vi "UHR-Fleezers Control (host) - 12.0_test_fpga_connection.vi"() -> ()   [LabVIEW 2014] (continued)
                                n670 = case shown="False" w1010 {
                                tunnel: w1011 -> [_ w1040]
                                tunnel: w1009 -> [w1012 _]
                                frame False {
                                n671 = flat-sequence {
                                tunnel: w1012 -> [w1013]
                                frame #0 {
                                n672 = property on="Trap Pos FB SP" class="DigNum (strict)"("Val(Sgnl)"=w1013) -> ()  [unwired: 2 in, 2 out]
                                }
                                frame #1 {
                                n673 = Wait (ms)(milliseconds to wait=u32 700) -> ()  [unwired: 1 out]
                                }
                                frame #2 {
                                n674 = local read "Action (%)"() -> (w1018:dbl)
                                n675 = Absolute Value(x=w1018) -> (abs(x)=w1017:dbl)
                                n676 = Greater?(x=w1017, y=70.0) -> (0:w1015:bool)
                                n677 = property on="Remove Action Offset" class="Bool (strict)"("Val(Sgnl)"=w1015) -> ()  [unwired: 2 in, 2 out]
                                }
                                frame #3 {
                                n678 = for {
                                N: 4 -> [_]
                                n679 = flat-sequence {
                                frame #0 {
                                n680 = Wait (ms)(milliseconds to wait=u32 500) -> ()  [unwired: 1 out]
                                }
                                frame #1 {
                                n681 = local read "Action (%)"() -> (w1024:dbl)
                                n682 = Absolute Value(x=w1024) -> (abs(x)=w1023:dbl)
                                n683 = Greater?(x=w1023, y=70.0) -> (0:w1021:bool)
                                n684 = property on="Remove Action Offset" class="Bool (strict)"("Val(Sgnl)"=w1021) -> ()  [unwired: 2 in, 2 out]
                                }
                                }
                                }
                                }
                                frame #4 {
                                n685 = Wait (ms)(milliseconds to wait=u32 500) -> ()  [unwired: 1 out]
                                }
                                frame #5 {
                                n686 = local read "Shift confocal"() -> (w1029:bool)
                                n687 = local read "Mean"() -> (w1032:dbl)
                                n688 = Greater?(x=w1032, y=11.0) -> (0:w1028:bool)
                                n689 = Not(x=w1028) -> (.not. x?=w1027:bool)
                                n690 = And(x=w1028, y=w1029) -> (x .and. y?=w1030:bool)
                                n691 = And(x=w1027, y=w1029) -> (x .and. y?=w1026:bool)
                                n692 = case shown="True" w1030 {
                                frame False {
                                }
                                frame True {
                                n693 = local read "Confocal X 2 (V)"() -> (w1035:dbl)
                                n694 = local read "Confocal Y 2 (V)"() -> (w1036:dbl)
                                n695 = property on="AO2" class="Slide (strict)"("Val(Sgnl)"=w1035) -> ()  [unwired: 2 in, 2 out]
                                n696 = property on="AO1" class="Slide (strict)"("Val(Sgnl)"=w1036) -> ()  [unwired: 2 in, 2 out]
                                }
                                }
                                n697 = case shown="True" w1026 {
                                frame False {
                                }
                                frame True {
                                n698 = local read "Confocal Y 1 (V)"() -> (w1034:dbl)
                                n699 = local read "Confocal X 1 (V)"() -> (w1033:dbl)
                                n700 = property on="AO1" class="Slide (strict)"("Val(Sgnl)"=w1034) -> ()  [unwired: 2 in, 2 out]
                                n701 = property on="AO2" class="Slide (strict)"("Val(Sgnl)"=w1033) -> ()  [unwired: 2 in, 2 out]
                                }
                                }
                                }
                                frame #6 {
                                n702 = Wait (ms)(milliseconds to wait=u32 1500) -> ()  [unwired: 1 out]
                                }
                                frame #7 {
                                n703 = property on="Remove Offset" class="Bool (strict)"("Val(Sgnl)"=TRUE ("Value (Signaling)")) -> ()  [unwired: 2 in, 2 out]
                                n704 = property on="Rem fb disp offset" class="Bool (strict)"("Val(Sgnl)"=TRUE ("Value (Signaling)")) -> ()  [unwired: 2 in, 2 out]
                                }
                                }
                                }
                                frame True {
                                n705 = flat-sequence {
                                tunnel: w1040 -> [w1041]
                                frame #0 {
                                n706 = property on="Trap D (MHz)" class="DigNum (strict)"("Val(Sgnl)"=w1041) -> ()  [unwired: 2 in, 2 out]
                                }
                                frame #1 {
                                n707 = Wait (ms)(milliseconds to wait=u32 500) -> ()  [unwired: 1 out]
                                }
                                frame #2 {
                                n708 = local read "Shift confocal"() -> (w1047:bool)
                                n709 = local read "Mean"() -> (w1048:dbl)
                                n710 = Greater?(x=w1048, y=11.0) -> (0:w1046:bool)
                                n711 = And(x=w1046, y=w1047) -> (x .and. y?=w1044:bool)
                                n712 = Not(x=w1046) -> (.not. x?=w1045:bool)
                                n713 = And(x=w1045, y=w1047) -> (x .and. y?=w1043:bool)
                                n714 = case shown="True" w1044 {
                                frame False {
                                }
                                frame True {
                                n715 = local read "Confocal Y 2 (V)"() -> (w1053:dbl)
                                n716 = local read "Confocal X 2 (V)"() -> (w1052:dbl)
                                n717 = property on="AO1" class="Slide (strict)"("Val(Sgnl)"=w1053) -> ()  [unwired: 2 in, 2 out]
                                n718 = property on="AO2" class="Slide (strict)"("Val(Sgnl)"=w1052) -> ()  [unwired: 2 in, 2 out]
                                }
                                }
                                n719 = case shown="True" w1043 {
                                frame False {
                                }
                                frame True {
                                n720 = local read "Confocal Y 1 (V)"() -> (w1051:dbl)
                                n721 = local read "Confocal X 1 (V)"() -> (w1050:dbl)
                                n722 = property on="AO2" class="Slide (strict)"("Val(Sgnl)"=w1050) -> ()  [unwired: 2 in, 2 out]
                                n723 = property on="AO1" class="Slide (strict)"("Val(Sgnl)"=w1051) -> ()  [unwired: 2 in, 2 out]
                                }
                                }
                                }
                                }
                                }
                                }
                                }
                                }
                                }
                                }
                                n724 = local read "Time (s)"() -> (w987:dbl)
                                n725 = Subtract(x=w988, y=w987) -> (x-y=w999:dbl)
                                n726 = Number To Decimal String(number=w999, width (-)=i16 0) -> (decimal integer string=w997:string)
                                n727 = Concatenate Strings(w997, " s fluorescence event") -> (w994:string)
                                n728 = local read "Messages"() -> (w995:string)
                                n729 = local write "Duration (s)"(w999) -> ()
                                n730 = call "Update messages.vi"("Message to add"=w994, "Old message string"=w995) -> ("New message string"=w993:string)
                                n731 = local write "Messages"(w993) -> ()
                                n732 = call <vilib>:"Beep.vi"() -> ()  [unwired: 12 in]
                                n733 = local write "Reset Force"(FALSE ("Force Reset")) -> ()
                                n734 = local write "Fl. High"(TRUE ("Fl. High")) -> ()
                                n735 = local write "Waiting"(TRUE ("Waiting")) -> ()
                                }
                                }
                                n736 = node-c288() -> ()  [unwired: 1 in, 1 out]
                                }
                                n737 = node-c288(w966) -> ()  [unwired: 1 out]
                                }
                              }
                            }
                          }
                          n738 = local read "Trap Pos FB SP"() -> (w875:fxp<+/-,16,1>)
                          n739 = local read "Trap D (MHz)"() -> (w877:dbl)
                        }
                      }
                    }
                    frame True {
                      n740 = flat-sequence {
                        tunnel: w1064 -> [w1074]
                        tunnel: [w1074] -> w1068
                        tunnel: w1067 -> [w1073]
                        tunnel: [w1073] -> w1066
                        tunnel: [w1072] -> w1065
                        tunnel: w1063 -> [w1071]
                        tunnel: [w1070] -> w1062
                        tunnel: w1059 -> [w1069]
                        tunnel: [w1069] -> w1058
                        tunnel: w1068 -> [w1146]
                        tunnel: w1066 -> [w1145]
                        tunnel: w1065 -> [w1144]
                        tunnel: w1062 -> [w1143]
                        tunnel: w1058 -> [w1142]
                        tunnel: [w1143] -> w1061
                        frame #0 {
                          n741 = call <vilib>:"Beep.vi"() -> ()  [unwired: 3 in, 9 out]
                          n742 = local write "Waiting"(FALSE ("Waiting")) -> ()
                          n743 = Increment(x=w1071) -> (x+1=w1070:u8)
                          n744 = case shown="\"Image\"" w1073 {
                            tunnel: w1070 -> [_ _ w1080 _]
                            frame "Image" {
                              n745 = property on="Confocal\nImage" class="Bool (strict)"("Val(Sgnl)"=TRUE ("Value (Signaling)")) -> ()  [unwired: 2 in, 2 out]
                            }
                            frame "Alarm", Default {
                            }
                            frame "Yank" {
                              n746 = flat-sequence {
                                tunnel: w1080 -> [w1083]
                                tunnel: [w1082] -> w1079
                                tunnel: ["N Array El"] -> w1078
                                tunnel: w1079 -> [w1097]
                                tunnel: w1078 -> [w1093]
                                frame #0 {
                                n747 = Multiply(x="Yank Delay (s)", y=1000.0) -> (x*y=w1086:dbl)
                                n748 = Quotient & Remainder(x=w1083, y="N Array El") -> (x-y*floor(x/y)=w1082:u8)  [unwired: 1 out]
                                n749 = Wait (ms)(milliseconds to wait=w1086) -> ()  [unwired: 1 out]
                                }
                                frame #1 {
                                n750 = Random Number (0-1)() -> (number: 0 to 1=w1094:dbl)
                                n751 = Multiply(x=w1093, y=w1094) -> (x*y=w1092:dbl)
                                n752 = Round Toward -Infinity(1:w1092) -> (0:w1091:dbl)
                                n753 = Select(t=w1091, s="Random Choice", f=w1097) -> (s? t:f=w1095:dbl)
                                n754 = Select(t="Yank to Trap D (MHz)", s="Yank to which?", f="Yank to SP") -> (s? t:f=w1088:dbl[])
                                n755 = Index Array(array=w1088, index=w1095) -> (element=w1098:dbl)
                                n756 = case shown="False" "Yank to which?" {
                                tunnel: w1098 -> [w1099 w1126]
                                frame False {
                                n757 = flat-sequence {
                                tunnel: w1099 -> [w1100]
                                frame #0 {
                                n758 = property on="Trap Pos FB SP" class="DigNum (strict)"("Val(Sgnl)"=w1100) -> ()  [unwired: 2 in, 2 out]
                                }
                                frame #1 {
                                n759 = Wait (ms)(milliseconds to wait=u32 700) -> ()  [unwired: 1 out]
                                }
                                frame #2 {
                                n760 = local read "Action (%)"() -> (w1105:dbl)
                                n761 = Absolute Value(x=w1105) -> (abs(x)=w1104:dbl)
                                n762 = Greater?(x=w1104, y=70.0) -> (0:w1102:bool)
                                n763 = property on="Remove Action Offset" class="Bool (strict)"("Val(Sgnl)"=w1102) -> ()  [unwired: 2 in, 2 out]
                                }
                                frame #3 {
                                n764 = for {
                                N: 4 -> [_]
                                n765 = flat-sequence {
                                frame #0 {
                                n766 = Wait (ms)(milliseconds to wait=u32 500) -> ()  [unwired: 1 out]
                                }
                                frame #1 {
                                n767 = local read "Action (%)"() -> (w1111:dbl)
                                n768 = Absolute Value(x=w1111) -> (abs(x)=w1110:dbl)
                                n769 = Greater?(x=w1110, y=70.0) -> (0:w1108:bool)
                                n770 = property on="Remove Action Offset" class="Bool (strict)"("Val(Sgnl)"=w1108) -> ()  [unwired: 2 in, 2 out]
                                }
                                }
                                }
                                }
                                frame #4 {
                                n771 = local read "Shift confocal"() -> (w1115:bool)
                                n772 = local read "Mean"() -> (w1118:dbl)
                                n773 = Greater?(x=w1118, y=11.0) -> (0:w1114:bool)
                                n774 = Not(x=w1114) -> (.not. x?=w1113:bool)
                                n775 = And(x=w1113, y=w1115) -> (x .and. y?=w1112:bool)
                                n776 = And(x=w1114, y=w1115) -> (x .and. y?=w1116:bool)
                                n777 = case shown="True" w1116 {
                                frame False {
                                }
                                frame True {
                                n778 = local read "Confocal X 2 (V)"() -> (w1121:dbl)
                                n779 = local read "Confocal Y 2 (V)"() -> (w1122:dbl)
                                n780 = property on="AO2" class="Slide (strict)"("Val(Sgnl)"=w1121) -> ()  [unwired: 2 in, 2 out]
                                n781 = property on="AO1" class="Slide (strict)"("Val(Sgnl)"=w1122) -> ()  [unwired: 2 in, 2 out]
                                }
                                }
                                n782 = case shown="True" w1112 {
                                frame False {
                                }
                                frame True {
                                n783 = local read "Confocal X 1 (V)"() -> (w1119:dbl)
                                n784 = local read "Confocal Y 1 (V)"() -> (w1120:dbl)
                                n785 = property on="AO1" class="Slide (strict)"("Val(Sgnl)"=w1120) -> ()  [unwired: 2 in, 2 out]
                                n786 = property on="AO2" class="Slide (strict)"("Val(Sgnl)"=w1119) -> ()  [unwired: 2 in, 2 out]
                                }
                                }
                                }
                                frame #5 {
                                n787 = Wait (ms)(milliseconds to wait=u32 1500) -> ()  [unwired: 1 out]
                                }
                                frame #6 {
                                n788 = property on="Remove Offset" class="Bool (strict)"("Val(Sgnl)"=TRUE ("Value (Signaling)")) -> ()  [unwired: 2 in, 2 out]
                                n789 = property on="Rem fb disp offset" class="Bool (strict)"("Val(Sgnl)"=TRUE ("Value (Signaling)")) -> ()  [unwired: 2 in, 2 out]
                                }
                                }
                                }
                                frame True {
                                n790 = flat-sequence {
                                tunnel: w1126 -> [w1127]
                                frame #0 {
                                n791 = property on="Trap D (MHz)" class="DigNum (strict)"("Val(Sgnl)"=w1127) -> ()  [unwired: 2 in, 2 out]
                                }
                                frame #1 {
                                n792 = Wait (ms)(milliseconds to wait=u32 500) -> ()  [unwired: 1 out]
                                }
                                frame #2 {
                                n793 = local read "Shift confocal"() -> (w1131:bool)
                                n794 = local read "Mean"() -> (w1129:dbl)
                                n795 = Greater?(x=w1129, y=11.0) -> (0:w1132:bool)
                                n796 = Not(x=w1132) -> (.not. x?=w1133:bool)
                                n797 = And(x=w1133, y=w1131) -> (x .and. y?=w1135:bool)
                                n798 = And(x=w1132, y=w1131) -> (x .and. y?=w1134:bool)
                                n799 = case shown="True" w1134 {
                                frame False {
                                }
                                frame True {
                                n800 = local read "Confocal Y 2 (V)"() -> (w1139:dbl)
                                n801 = local read "Confocal X 2 (V)"() -> (w1138:dbl)
                                n802 = property on="AO1" class="Slide (strict)"("Val(Sgnl)"=w1139) -> ()  [unwired: 2 in, 2 out]
                                n803 = property on="AO2" class="Slide (strict)"("Val(Sgnl)"=w1138) -> ()  [unwired: 2 in, 2 out]
                                }
                                }
                                n804 = case shown="True" w1135 {
                                frame False {
                                }
                                frame True {
                                n805 = local read "Confocal X 1 (V)"() -> (w1136:dbl)
                                n806 = local read "Confocal Y 1 (V)"() -> (w1137:dbl)
                                n807 = property on="AO2" class="Slide (strict)"("Val(Sgnl)"=w1136) -> ()  [unwired: 2 in, 2 out]
                                n808 = property on="AO1" class="Slide (strict)"("Val(Sgnl)"=w1137) -> ()  [unwired: 2 in, 2 out]
                                }
                                }
                                }
                                }
                                }
                                }
                                }
                              }
                            }
                            frame "Raster" {
                              n809 = property on="Trap Raster Scan" class="Bool (strict)"("Val(Sgnl)"=TRUE ("Value (Signaling)")) -> ()  [unwired: 2 in, 2 out]
                            }
                          }
                          n810 = local read "Time (s)"() -> (w1072:dbl)
                          "Fl. High" <- TRUE ("Yanking")
                        }
                        frame #1 {
                          n811 = local read "Auto F Reset"() -> (w1141:bool)
                          n812 = case shown="True" w1141 {
                            tunnel: w1146 -> [_ w1150]
                            tunnel: w1145 -> [_ w1149]
                            tunnel: w1144 -> [_ w1148]
                            tunnel: w1142 -> [_ w1147]
                            frame False {
                            }
                            frame True {
                              n813 = node-c288() -> (w1152:T26)  [unwired: 4 out]
                              n814 = timed-loop {
                                timing: w1152 -> [_]
                                timing-out: [_] -> w1151
                                tunnel: w1150 -> [w1170]
                                tunnel: w1149 -> [w1169]
                                tunnel: w1148 -> [w1168]
                                tunnel: w1147 -> [w1167]
                                stop <- w1153 stop-if-true
                                n815 = node-c288() -> ()  [unwired: 2 out]
                                n816 = local read "Fl. D Thresh. (kHz)"() -> (w1161:dbl)
                                n817 = local read "Fl. Triggered..."() -> (w1166:bool)
                                n818 = local read "Delta Fl. 1"() -> (w1157:dbl)
                                n819 = local read "Delta Fl. 2"() -> (w1155:dbl)
                                n820 = local read "Stop All"() -> (w1164:bool)
                                n821 = local read "APD to Watch"() -> (w1156:bool)
                                n822 = Select(t=w1157, s=w1156, f=w1155) -> (s? t:f=w1154:dbl)
                                n823 = Not(x=w1166) -> (.not. x?=w1165:bool)
                                n824 = Multiply(x=w1161, y=1000.0) -> (x*y=w1160:dbl)
                                n825 = Negate(x=w1160) -> (-x=w1159:dbl)
                                n826 = Less?(x=w1154, y=w1159) -> (x < y?=w1163:bool)
                                n827 = Compound Arithmetic op=OR(w1163, w1164, w1165, "Reset Force") -> (w1153:bool)
                                n828 = case shown="True" w1153 {
                                tunnel: w1170 -> [_ w1185]
                                tunnel: w1169 -> [_ w1184]
                                tunnel: w1168 -> [_ w1174]
                                tunnel: w1167 -> [_ w1176]
                                frame False {
                                }
                                frame True {
                                n829 = local read "Time (s)"() -> (w1175:dbl)
                                n830 = case shown="\"Yank\"" w1184 {
                                tunnel: w1185 -> [_ w1188]
                                tunnel: w1176 -> [_ w1186]
                                frame "Image", Default {
                                }
                                frame "Yank" {
                                n831 = flat-sequence {
                                tunnel: [w1194] -> w1189
                                tunnel: w1188 -> [w1194]
                                tunnel: [w1190] -> w1187
                                tunnel: w1186 -> [w1190]
                                tunnel: w1189 -> [w1197]
                                tunnel: w1187 -> [w1195]
                                frame #0 {
                                n832 = local read "Yank Delay (s)"() -> (w1193:dbl)
                                n833 = Multiply(x=w1193, y=1000.0) -> (x*y=w1191:dbl)
                                n834 = Wait (ms)(milliseconds to wait=w1191) -> ()  [unwired: 1 out]
                                }
                                frame #1 {
                                n835 = local read "Yank to which?"() -> (w1196:bool)
                                n836 = case shown="False" w1196 {
                                tunnel: w1197 -> [_ w1225]
                                tunnel: w1195 -> [w1198 _]
                                frame False {
                                n837 = flat-sequence {
                                tunnel: w1198 -> [w1199]
                                frame #0 {
                                n838 = property on="Trap Pos FB SP" class="DigNum (strict)"("Val(Sgnl)"=w1199) -> ()  [unwired: 2 in, 2 out]
                                }
                                frame #1 {
                                n839 = Wait (ms)(milliseconds to wait=u32 700) -> ()  [unwired: 1 out]
                                }
                                frame #2 {
                                n840 = local read "Action (%)"() -> (w1204:dbl)
                                n841 = Absolute Value(x=w1204) -> (abs(x)=w1203:dbl)
                                n842 = Greater?(x=w1203, y=70.0) -> (0:w1201:bool)
                                n843 = property on="Remove Action Offset" class="Bool (strict)"("Val(Sgnl)"=w1201) -> ()  [unwired: 2 in, 2 out]
                                }
                                frame #3 {
                                n844 = for {
                                N: 4 -> [_]
                                n845 = flat-sequence {
                                frame #0 {
                                n846 = Wait (ms)(milliseconds to wait=u32 500) -> ()  [unwired: 1 out]
                                }
                                frame #1 {
                                n847 = local read "Action (%)"() -> (w1210:dbl)
                                n848 = Absolute Value(x=w1210) -> (abs(x)=w1209:dbl)
                                n849 = Greater?(x=w1209, y=70.0) -> (0:w1207:bool)
                                n850 = property on="Remove Action Offset" class="Bool (strict)"("Val(Sgnl)"=w1207) -> ()  [unwired: 2 in, 2 out]
                                }
                                }
                                }
                                }
                                frame #4 {
                                n851 = local read "Shift confocal"() -> (w1215:bool)
                                n852 = local read "Mean"() -> (w1217:dbl)
                                n853 = Greater?(x=w1217, y=11.0) -> (0:w1214:bool)
                                n854 = Not(x=w1214) -> (.not. x?=w1213:bool)
                                n855 = And(x=w1214, y=w1215) -> (x .and. y?=w1212:bool)
                                n856 = And(x=w1213, y=w1215) -> (x .and. y?=w1211:bool)
                                n857 = case shown="True" w1212 {
                                frame False {
                                }
                                frame True {
                                n858 = local read "Confocal Y 2 (V)"() -> (w1221:dbl)
                                n859 = local read "Confocal X 2 (V)"() -> (w1220:dbl)
                                n860 = property on="AO2" class="Slide (strict)"("Val(Sgnl)"=w1220) -> ()  [unwired: 2 in, 2 out]
                                n861 = property on="AO1" class="Slide (strict)"("Val(Sgnl)"=w1221) -> ()  [unwired: 2 in, 2 out]
                                }
                                }
                                n862 = case shown="True" w1211 {
                                frame False {
                                }
                                frame True {
                                n863 = local read "Confocal X 1 (V)"() -> (w1218:dbl)
                                n864 = local read "Confocal Y 1 (V)"() -> (w1219:dbl)
                                n865 = property on="AO1" class="Slide (strict)"("Val(Sgnl)"=w1219) -> ()  [unwired: 2 in, 2 out]
                                n866 = property on="AO2" class="Slide (strict)"("Val(Sgnl)"=w1218) -> ()  [unwired: 2 in, 2 out]
                                }
                                }
                                }
                                frame #5 {
                                n867 = Wait (ms)(milliseconds to wait=u32 1500) -> ()  [unwired: 1 out]
                                }
                                frame #6 {
                                n868 = property on="Rem fb disp offset" class="Bool (strict)"("Val(Sgnl)"=TRUE ("Value (Signaling)")) -> ()  [unwired: 2 in, 2 out]
                                n869 = property on="Remove Offset" class="Bool (strict)"("Val(Sgnl)"=TRUE ("Value (Signaling)")) -> ()  [unwired: 2 in, 2 out]
                                }
                                }
                                }
                                frame True {
                                n870 = flat-sequence {
                                tunnel: w1225 -> [w1226]
                                frame #0 {
                                n871 = property on="Trap D (MHz)" class="DigNum (strict)"("Val(Sgnl)"=w1226) -> ()  [unwired: 2 in, 2 out]
                                }
                                frame #1 {
                                n872 = Wait (ms)(milliseconds to wait=u32 500) -> ()  [unwired: 1 out]
                                }
                                frame #2 {
                                n873 = local read "Shift confocal"() -> (w1232:bool)
                                n874 = local read "Mean"() -> (w1234:dbl)
                                n875 = Greater?(x=w1234, y=11.0) -> (0:w1231:bool)
                                n876 = Not(x=w1231) -> (.not. x?=w1230:bool)
                                n877 = And(x=w1231, y=w1232) -> (x .and. y?=w1229:bool)
                                n878 = And(x=w1230, y=w1232) -> (x .and. y?=w1228:bool)
                                n879 = case shown="True" w1229 {
                                frame False {
                                }
                                frame True {
                                n880 = local read "Confocal Y 2 (V)"() -> (w1238:dbl)
                                n881 = local read "Confocal X 2 (V)"() -> (w1237:dbl)
                                n882 = property on="AO2" class="Slide (strict)"("Val(Sgnl)"=w1237) -> ()  [unwired: 2 in, 2 out]
                                n883 = property on="AO1" class="Slide (strict)"("Val(Sgnl)"=w1238) -> ()  [unwired: 2 in, 2 out]
                                }
                                }
                                n884 = case shown="True" w1228 {
                                frame False {
                                }
                                frame True {
                                n885 = local read "Confocal Y 1 (V)"() -> (w1236:dbl)
                                n886 = local read "Confocal X 1 (V)"() -> (w1235:dbl)
                                n887 = property on="AO2" class="Slide (strict)"("Val(Sgnl)"=w1235) -> ()  [unwired: 2 in, 2 out]
                                n888 = property on="AO1" class="Slide (strict)"("Val(Sgnl)"=w1236) -> ()  [unwired: 2 in, 2 out]
                                }
                                }
                                }
                                }
                                }
                                }
                                }
                                }
                                }
                                }
                                n889 = local read "Messages"() -> (w1183:string)
                                n890 = Subtract(x=w1175, y=w1174) -> (x-y=w1181:dbl)
                                "Duration (s)" <- w1181
                                n891 = Number To Decimal String(number=w1181, width (-)=i16 0) -> (decimal integer string=w1179:string)
                                n892 = Concatenate Strings(w1179, " s fluorescence event." ("string")) -> (w1177:string)
                                n893 = call "Update messages.vi"("Message to add"=w1177, "Old message string"=w1183) -> ("New message string"=w1182:string)
                                n894 = local write "Reset Force"(FALSE ("Reset Force")) -> ()
                                n895 = local write "Waiting"(TRUE ("Waiting")) -> ()
                                n896 = local write "Messages"(w1182) -> ()
                                n897 = local write "Fl. High"(FALSE ("Fl. High")) -> ()
                                n898 = call <vilib>:"Beep.vi"() -> ()  [unwired: 3 in, 9 out]
                                }
                                }
                                n899 = node-c288() -> ()  [unwired: 2 out]
                              }
                              n900 = node-c288(w1151) -> ()  [unwired: 1 out]
                            }
                          }
                        }
                      }
                      n901 = local read "Trap Pos FB SP"() -> (w1059:fxp<+/-,16,1>)
                      n902 = local read "Trap D (MHz)"() -> (w1064:dbl)
                    }
                  }
                }
                frame #1 {
                  n903 = local read "Stop All"() -> (w1248:bool)
                  n904 = local read "Fl. Triggered..."() -> (w1246:bool)
                  n905 = Not(x=w1246) -> (.not. x?=w1247:bool)
                  n906 = Or(x=w1247, y=w1248) -> (x .or. y?=w1245:bool)
                }
              }
              n907 = case shown="True" w834 {
                frame False {
                }
                frame True {
                  n908 = local read "Confocal Y 1 (V)"() -> (w844:dbl)
                  n909 = local read "Confocal X 1 (V)"() -> (w843:dbl)
                  n910 = property on="AO2" class="Slide (strict)"("Val(Sgnl)"=w843) -> ()  [unwired: 2 in, 2 out]
                  n911 = property on="AO1" class="Slide (strict)"("Val(Sgnl)"=w844) -> ()  [unwired: 2 in, 2 out]
                }
              }
              n912 = case shown="True" w834 {
                frame False {
                }
                frame True {
                  w842 = FALSE ("Fl. High")
                  n913 = local write "Waiting"(w842) -> ()
                  n914 = local write "Fl. High"(w842) -> ()
                }
              }
              n915 = node-c288() -> ()  [unwired: 2 out]
            }
            n916 = node-c288(w832) -> ()  [unwired: 1 out]
          }
        }
      }
      event "Stop All": Value Change {
        n917 = event-data() -> ()  [unwired: 7 out]
        n918 = local read "Stop All"() -> (w1253:bool)
      }
    }
    n919 = node-c288() -> ()  [unwired: 2 out]
  }
  n920 = property on="Saved trap pos" class="WFGraph (strict)"("Visible"=TRUE) -> ()  [unwired: 2 in, 2 out]
  n921 = property on="Trap Delta Graph" class="WFGraph (strict)"("Visible"=FALSE) -> ()  [unwired: 2 in, 2 out]
  n922 = local write "Trap pos"(TRUE ("Trap pos")) -> ()
  n923 = node-c288(2 ("Processor")) -> (w137:T26)  [unwired: 3 out]
  n924 = timed-loop "Control parameters (event loop)" {
    tunnel: w51 -> [w1262]
    shift-right: [w1261] -> _
    shift-left: errorcluster {"status"=FALSE, "code"=0, "source"=""} ("error out") -> [w1260]
    tunnel: [w1259] -> _
    timing: w137 -> [_]
    timing-out: [_] -> w136
    tunnel: w111 -> [w1258]
    tunnel: w55 -> [w1257]
    tunnel: w54 -> [w1256]
    tunnel: w53 -> [w1255]
    tunnel: w52 -> [w1254]
    stop <- w1259 stop-if-true
    n925 = node-c288() -> ()  [unwired: 2 out]
    n926 = event shown="[77] \"Save user params\": Value Change" {
      selector: _ -> [_ _ _ _ _ _ _ _ _ _ _ _ _ _ _ _ _ _ _ _ _ _ _ _ _ _ _ _ _ _ _ _ _ _ _ _ _ _ _ _ _ _ _ _ _ _ _ _ _ _ _ _ _ _ _ _ _ _ _ _ _ _ _ _ _ _ _ _ _ _ _ _ _ _ _ _ _ _ _ _]
      dyn-events: _ -> [_ _ _ _ _ _ _ _ _ _ _ _ _ _ _ _ _ _ _ _ _ _ _ _ _ _ _ _ _ _ _ _ _ _ _ _ _ _ _ _ _ _ _ _ _ _ _ _ _ _ _ _ _ _ _ _ _ _ _ _ _ _ _ _ _ _ _ _ _ _ _ _ _ _ _ _ _ _ _ _]
      timeout: _ -> [_ _ _ _ _ _ _ _ _ _ _ _ _ _ _ _ _ _ _ _ _ _ _ _ _ _ _ _ _ _ _ _ _ _ _ _ _ _ _ _ _ _ _ _ _ _ _ _ _ _ _ _ _ _ _ _ _ _ _ _ _ _ _ _ _ _ _ _ _ _ _ _ _ _ _ _ _ _ _ _]
      tunnel: w1262 -> [w1300 _ _ _ w1338 _ w1360 _ _ _ _ w1426 _ _ w1469 w1475 w1480 w1486 w1522 w1549 w1559 _ w1578 w1582 w1593 w1604 w1615 w1632 w1643 w1654 w1681 w1775 w1782 w1820 _ _ w1880 w1884 w1895 w1899 w1903 _ w1911 _ _ _ _ _ _ _ _ _ _ _ _ _ _ _ _ _ w2292 _ w2309 _ w2316 w2334 _ w2341 w2349 w2364 w2375 w2381 _ w2390 _ w2409 _ _ _ w2484]
      tunnel: [w1299 _ _ _ w1328 _ w1359 _ _ w1391 _ w1405 _ _ w1468 w1471 w1477 w1483 w1521 w1547 w1558 _ w1576 _ w1587 w1598 w1609 w1626 w1637 w1648 w1679 w1773 w1780 w1818 _ _ w1878 w1882 w1885 w1897 w1901 _ w1909 _ _ _ _ _ _ _ _ _ _ _ _ _ _ _ _ _ w2290 _ _ _ _ w2331 _ _ _ _ _ _ _ _ _ _ _ _ _ w2482] -> w1261
      tunnel: w1260 -> [w1298 _ _ _ w1337 _ w1358 _ _ w1391 _ w1425 _ _ w1467 w1470 w1476 w1482 w1520 w1548 w1557 _ w1577 w1581 w1592 w1603 w1614 w1631 w1642 w1653 w1680 w1774 w1781 w1819 _ _ w1879 w1883 w1894 w1898 w1902 _ w1910 _ _ _ _ _ _ _ _ _ _ _ _ _ _ _ _ _ w2291 _ w2308 _ w2315 w2333 _ w2340 w2348 w2363 w2374 w2380 _ w2389 _ w2408 _ _ _ w2483]
      tunnel: [_ _ _ _ _ _ _ _ _ w1390 _ _ _ _ _ _ _ _ _ _ _ _ _ _ _ _ _ _ _ _ _ _ _ _ _ _ _ _ _ _ _ _ _ _ _ _ _ _ _ _ _ _ _ _ _ _ _ _ _ _ _ _ _ _ _ _ _ _ _ _ _ _ _ _ _ _ _ _ _ _] -> w1259
      tunnel: [_ _ _ _ _ _ _ "Round T1 X" _ _ _ _ _ _ _ _ _ _ _ _ _ _ _ _ _ _ _ _ _ _ _ _ _ _ _ _ _ _ _ _ _ _ _ _ _ _ _ _ _ _ _ _ _ _ _ _ _ _ _ _ _ _ _ _ _ _ _ _ _ _ _ _ _ _ _ _ _ _ _ _] -> _
      tunnel: [_ _ _ "Adjust Scale\nto Mean" _ _ _ _ _ _ _ _ _ _ _ _ _ _ _ _ _ _ "Test ttrig" _ _ _ _ _ _ _ _ _ _ _ _ _ _ _ _ _ _ _ _ _ _ _ _ _ _ _ "Flush Sample" "Flush Pump 3" "Flush Pump 1" "Clear Volume" _ _ _ _ _ _ _ _ _ _ _ _ _ _ _ _ _ _ _ _ _ _ _ _ _ _] -> _
      tunnel: [_ _ _ _ _ _ _ _ "Round T2 X" _ "Delayed Interlace Start" _ _ _ _ _ _ _ _ _ _ _ _ _ _ _ _ _ _ _ _ _ _ _ _ _ _ _ _ _ _ _ _ _ _ _ _ _ _ _ _ _ _ _ _ _ _ _ _ _ _ _ _ _ _ _ _ _ _ _ _ _ _ _ _ _ _ _ _ _] -> _
      tunnel: w1258 -> [_ _ _ _ _ _ _ _ _ _ _ _ _ _ _ _ _ _ _ _ _ _ _ _ _ _ _ _ _ _ _ _ _ _ _ _ _ _ _ _ _ _ _ _ _ _ w2069 w2087 w2094 w2099 w2105 _ _ w2204 _ _ _ _ _ _ _ _ _ _ _ _ _ _ _ _ _ _ _ _ _ _ _ _ _ _]
      tunnel: w1257 -> [_ _ _ _ _ _ _ _ _ _ _ _ _ _ _ _ _ _ _ _ _ _ _ _ _ _ _ _ _ _ _ _ _ _ _ _ _ _ _ _ _ _ _ _ w1985 _ _ _ _ _ _ w2135 _ _ w2211 _ w2220 _ w2234 _ _ _ _ _ _ _ _ _ _ _ _ _ _ _ _ _ _ _ _ _]
      tunnel: w1256 -> [_ _ _ _ _ _ _ _ _ _ _ _ _ _ _ _ _ _ _ _ _ _ _ _ _ _ _ _ _ _ _ _ _ _ _ _ _ _ _ _ _ _ _ _ _ _ _ _ _ _ _ _ _ _ _ _ _ _ _ _ _ _ _ _ _ _ _ _ _ _ _ _ _ _ _ _ _ _ _ _]
      tunnel: w1255 -> [_ _ _ _ _ _ _ _ _ _ _ _ _ _ _ _ _ _ _ _ _ _ _ _ _ _ _ _ _ _ _ _ _ _ _ _ _ _ _ _ _ _ _ w1922 _ _ _ _ _ _ _ _ w2165 _ _ w2216 _ w2227 _ w2259 _ _ _ _ _ _ _ _ _ _ _ _ _ _ _ _ _ _ _ _]
      tunnel: w1254 -> [_ _ _ _ _ _ _ _ _ _ _ _ _ _ _ _ _ _ _ _ _ _ _ _ _ _ _ _ _ _ _ _ _ _ _ _ _ _ _ _ _ _ _ _ _ _ _ _ _ _ _ _ _ _ _ _ _ _ _ _ _ _ _ _ _ _ _ _ _ _ _ _ _ _ _ _ _ _ _ _]
      event "AI Count (ticks)", "Sets to FIFO (Traps)", "Save ave N", "FPGA Ave.", "# Samples/channel", "N sets to save": Value Change {
        # "So that if 'Save ave N' is updated, the AOD scanning code updates too."
        n927 = event-data() -> ()  [unwired: 6 out]
        n928 = local read "AI Count (ticks)"() -> (w1280:u32)
        n929 = Boolean To (0,1)(Boolean="Sets to FIFO (Traps)") -> (0, 1=w1290:cluster{"Set 1":i16, "Set 2":i16, "Set 3":i16})
        n930 = Cluster To Array(cluster=w1290) -> (array=w1289:i16[])
        n931 = xnode "Read/Write Control"("FPGA VI Reference In"=w1300, "error in"=w1298, "ai count"=w1280, "AI1 Sets to FIFO"="Sets to FIFO (Traps)", "N of AI1 Int Acq Sets"="N Acq Sets (Traps + Fl.)") -> ("error out"=w1299:errorcluster)  [unwired: 1 out]
        n932 = To Unsigned Long Integer(number=w1289) -> (unsigned 32bit integer=w1269:u32[])
        n933 = local read "Scan steps (AOD)"() -> (w1291:u64)
        n934 = Multiply(x=w1280, y="N Acq Sets (Traps + Fl.)") -> (x*y=w1278:u32)
        n935 = Divide(x=40000000.0, y=w1280) -> (x/y=w1272:dbl)
        "AI rate (Hz)" <- w1272
        "Ave. Rate (Hz)" <- w1272
        n936 = Add Array Elements(numeric array=w1269) -> (sum=w1281:u32)
        "Trap Sets" <- w1281
        n937 = Reciprocal(x=w1272) -> (1/x=→"Ave. Period (s)":dbl)
        n938 = property on="Scan steps (AOD)" class="DigNum (strict)"("Val(Sgnl)"=w1291) -> ()  [unwired: 2 in, 2 out]
        n939 = Divide(x=w1272, y="N Acq Sets (Traps + Fl.)") -> (x/y=w1295:dbl)
        "Data Rate (Hz)" <- w1295
        n940 = Reciprocal(x=w1295) -> (1/x=→"Data Period (s)":dbl)
        n941 = local read "Save ave N"() -> (w1294:dbl)
        n942 = Divide(x=w1295, y=w1294) -> (x/y=w1293:dbl)
        "Save Data Rate (Hz)" <- w1293
        n943 = Reciprocal(x=w1293) -> (1/x=→"Save Data Period (s)":dbl)
        n944 = Multiply(x=w1278, y="# Samples/trap") -> (x*y=w1276:u32)
        "Counts/DMA" <- w1276
        n945 = property on="Trap Disp. Downsample" class="DigNum (strict)"("Maximum"="# Samples/trap") -> ()  [unwired: 2 in, 2 out]
        n946 = Multiply(x=w1281, y="# Samples/trap") -> (x*y=w1270:u32)
        "# Samples/channel" <- w1270
        n947 = Multiply(x=w1270, y=u32 8) -> (x*y=→"Trap AI Elements/DMA read":u32)
        n948 = local read "APD Int. Count"() -> (w1277:u32)
        n949 = Multiply(x=w1270, y=u32 3) -> (x*y=→"Trap Pos Elements/DMA read":u32)
        n950 = Divide(x=w1276, y=w1277) -> (x/y=w1267:dbl)
        "APD Samples/FIFO Acq." <- w1267
        n951 = Divide(x=w1276, y=40000000.0) -> (x/y=w1274:dbl)
        "DMA Update Period (s)" <- w1274
        n952 = Multiply(x=2.0, y=w1267) -> (x*y=→"APD Elements/DMA read":dbl)
        n953 = property on="APD Disp. Downsample" class="DigNum (strict)"("Maximum"=w1267) -> ()  [unwired: 2 in, 2 out]
        n954 = local read "N sets to save"() -> (w1287:u32)
        n955 = Multiply(x=w1274, y=w1287) -> (x*y=→"Total Time (s)":dbl)
        "FPGA Averaging" <- FALSE ("FPGA Averaging")
      }
      event "Remove Offset": Value Change {
        n956 = event-data() -> ()  [unwired: 7 out]
        n957 = local write "Remove Offset"(FALSE ("Remove Offset")) -> ()
        n958 = local read "Bead Mean (nm)"() -> (w1302:dbl)
        n959 = local read "Offset (nm)"() -> (w1303:dbl)
        n960 = Add(x=w1302, y=w1303) -> (x+y=w1301:dbl)
        n961 = local write "Offset (nm)"(w1301) -> ()
        n962 = disable-structure shown="Disabled" {
          frame Disabled {
            n963 = local read "Bead Mean (nm)"() -> (w1308:dbl)
            n964 = Add(y=w1308) -> (x=w1307:dbl, x+y=w1306:dbl)
            n965 = Subtract(x=w1308, y=w1307) -> (x-y=w1305:dbl)
            n966 = property on="Bead Separation" class="WFChart (strict)"("YScale.Minimum"=w1305) -> ()  [unwired: 2 in, 2 out]
            n967 = property on="Bead Separation" class="WFChart (strict)"("YScale.Maximum"=w1306) -> ()  [unwired: 2 in, 2 out]
          }
          frame Enabled {
          }
        }
      }
      event "Detector Type": Value Change {
        n968 = event-data() -> ()  [unwired: 7 out]
        n969 = local read "AI labels"() -> (w1309:string[])
        n970 = property on="High Res. Display" class="Ring (strict)"("Strings []"=w1309) -> ()  [unwired: 2 in, 2 out]
        n971 = Build Array (concatenate)(w1309, "none") -> (w1310:string[])
        n972 = property on="FFT 1 Choice 1" class="Ring (strict)"("Strings []"=w1310) -> ()  [unwired: 2 in, 2 out]
        n973 = property on="FFT 1 Choice 2" class="Ring (strict)"("Strings []"=w1310) -> ()  [unwired: 2 in, 2 out]
        n974 = property on="FFT 2 Choice 1" class="Ring (strict)"("Strings []"=w1310) -> ()  [unwired: 2 in, 2 out]
        n975 = property on="FFT 2 Choice 2" class="Ring (strict)"("Strings []"=w1310) -> ()  [unwired: 2 in, 2 out]
        n976 = Bundle("APD 1", "APD 2") -> (w1313:cluster{string, string})  [unwired: 1 out]
        n977 = Cluster To Array(cluster=w1313) -> (array=w1311:string[])
        n978 = Build Array (concatenate)(w1311, w1310) -> (w1315:string[])
        n979 = Array Size(array=w1315) -> (size(s)=w1316:i32)
        n980 = property on="Signals to Plot" class="LstBox (strict)"("Item Names"=w1315) -> ()  [unwired: 2 in, 2 out]
        n981 = property on="Signals to Plot" class="LstBox (strict)"("Number of Rows"=w1316) -> ()  [unwired: 2 in, 2 out]
        n982 = property on="All Signals" class="WFChart (strict)"("LegNumRows"=w1316) -> ()  [unwired: 2 in, 2 out]
      }
      event "Adjust Scale\nto Mean": Value Change {
        n983 = event-data() -> ()  [unwired: 7 out]
        n984 = local read "APD 1 Rate (Hz)"() -> (w1325:dbl)
        n985 = Multiply(x=1000.0, y="Above (kHz)") -> (x*y=w1323:dbl)
        n986 = Multiply(x=1000.0, y="Below (kHz)") -> (x*y=w1321:dbl)
        n987 = Add(x=w1323, y=w1325) -> (x+y=w1318:dbl)
        n988 = Subtract(x=w1325, y=w1321) -> (x-y=w1319:dbl)
        n989 = property on="APD Chart" class="WFChart (strict)"("YScale.Minimum"=w1319) -> ()  [unwired: 2 in, 2 out]
        n990 = property on="APD Chart" class="WFChart (strict)"("YScale.Maximum"=w1318) -> ()  [unwired: 2 in, 2 out]
      }
      event "Phase adj. (AI1)", "+ phase (AI1)", "- phase (AI1)": Value Change {
        n991 = event-data() -> ()  [unwired: 7 out]
        n992 = Negate(x="Phase adj. (AI1)") -> (-x=w1335:i16)
        n993 = Select(t=w1335, s="- phase (AI1)", f="Phase adj. (AI1)") -> (s? t:f=w1334:i16)
        n994 = xnode "Read/Write Control"("FPGA VI Reference In"=w1338, "error in"=w1337, "Phase count adjustment"=w1334) -> ("FPGA VI Reference Out"=w1333:T22, "error out"=w1332:errorcluster)
        n995 = Or(x="- phase (AI1)", y="+ phase (AI1)") -> (x .or. y?=w1329:bool)
        n996 = xnode "Read/Write Control"("FPGA VI Reference In"=w1333, "error in"=w1332, "+ phase"=w1329) -> ("error out"=w1328:errorcluster)  [unwired: 1 out]
      }
      event "Signals to Plot": Double Click {
        w1341 = u32 9868950 ("Color Box")
        n997 = event-data() -> ("Row"=w1343:i32)  [unwired: 9 out]
        n998 = property on="All Signals" class="WFChart (strict)"("Active Plot"=w1343) -> (error out=w1354:errorcluster)  [unwired: 2 in, 1 out]
        n999 = property on="All Signals" class="WFChart (strict)" props=["Plot", "Visible?", "Plot", "Plot Color"](error in=w1354) -> (error out=w1353:errorcluster, "Plot.Visible?"=w1352:bool)  [unwired: 1 in, 2 out]
        n1000 = Select(t=FALSE ("Plot.Visible"), s=w1352, f=TRUE ("Plot.Visible")) -> (s? t:f=w1347:bool)
        n1001 = property on="All Signals" class="WFChart (strict)"(error in=w1353, "Plot.Visible?"=w1347) -> (error out=w1349:errorcluster)  [unwired: 1 in, 1 out]
        n1002 = property on="All Signals" class="WFChart (strict)"(error in=w1349) -> (error out=w1344:errorcluster, "Plot.Plot Color"=w1348:u32)  [unwired: 1 in, 1 out]
        n1003 = property on="Signals to Plot" class="LstBox (strict)"(error in=w1344, "Active Row"=w1343) -> (error out=w1342:errorcluster)  [unwired: 1 in, 1 out]
        n1004 = Select(t=w1348, s=w1347, f=u32 0) -> (s? t:f=w1345:u32)
        n1005 = property on="Signals to Plot" class="LstBox (strict)"(error in=w1342, "CellFontColor"=w1345, "SelColor"=w1341, "CellBG"=w1341, "CellFontSize"=u32 20 ("Active Row:Cell Font:Size"), "CellFontBold"=TRUE ("Active Row:Cell Font:Bold")) -> ()  [unwired: 1 in, 2 out]
      }
      event "BD 1 Frequency 1 (MHz)", "BD 1 Frequency 2 (MHz)", "BD 1 Frequency 3 (MHz)", "BD 2 Frequency 1 (MHz)", "BD 2 Frequency 2 (MHz)", "BD 2 Frequency 3 (MHz)", "Trap D (MHz)": Value Change {
        n1006 = event-data() -> ("CtlRef"=w1357:refnum<vi>)  [unwired: 6 out]
        n1007 = control-ref of="Trap D (MHz)"() -> (w1356:refnum<vi>)
        n1008 = Equal?(x=w1356, y=w1357) -> (x = y?=w1355:bool)
        n1009 = case shown="False" "Oscillate Set 1" {
          tunnel: w1360 -> [w1380 _]
          tunnel: [w1379 w1383] -> w1359
          tunnel: w1358 -> [w1378 w1383]
          tunnel: w1355 -> [w1363 _]
          frame False {
            n1010 = local read "BD 1 Frequency 2 (MHz)"() -> (w1367:dbl)
            n1011 = local read "BD 1 Frequency 1 (MHz)"() -> (w1365:dbl)
            n1012 = Subtract(x=w1367, y="Trap D (MHz)") -> (x-y=w1364:dbl)
            n1013 = Select(t=w1364, s=w1363, f=w1365) -> (s? t:f=w1362:dbl)
            n1014 = local read "Y RF Frequency Limits (MHz)"() -> (w1368:T17)
            n1015 = local read "X RF Frequency Limits (MHz)"() -> (w1369:T17)
            n1016 = local read "BD 1 Frequency 3 (MHz)"() -> (w1381:dbl)
            n1017 = local write "BD 1 Frequency 1 (MHz)"(w1362) -> ()
            n1018 = local read "BD 2 Frequency 1 (MHz)"() -> (w1372:dbl)
            n1019 = local read "BD 2 Frequency 2 (MHz)"() -> (w1371:dbl)
            n1020 = local read "BD 2 Frequency 3 (MHz)"() -> (w1382:dbl)
            n1021 = call "set RF board frequency - interlace.vi"("Board 2 Frequency Limits"=w1368, "Board 1 Frequency Limits"=w1369, "error in"=w1378, "FPGA VI Reference In"=w1380, "Board 2 Frequency 3 (MHz)"=w1382, "Board 1 Frequency 3 (MHz)"=w1381, "Board 2 Frequency 2 (MHz)"=w1371, "Board 2 Frequency 1 (MHz)"=w1372, "Board 1 Frequency 2 (MHz)"=w1367, "Board 1 Frequency 1  (MHz)"=w1362) -> ("error out"=w1379:errorcluster)  [unwired: 1 out]
            n1022 = Subtract(x=w1372, y=w1371) -> (x-y=w1376:dbl)
            n1023 = Subtract(x=w1362, y=w1367) -> (x-y=w1377:dbl)
            n1024 = Square(x=w1376) -> (x^2=w1374:dbl)
            n1025 = Square(x=w1377) -> (x^2=w1375:dbl)
            n1026 = Add(x=w1375, y=w1374) -> (x+y=w1373:dbl)
            n1027 = Square Root(x=w1373) -> (sqrt(x)=w1370:dbl)
            n1028 = local write "Trap D (MHz)"(w1370) -> ()
            n1029 = property on="Initial D (MHz)" class="DigNum (strict)"("Val(Sgnl)"=w1370) -> ()  [unwired: 2 in, 2 out]
          }
          frame True {
          }
        }
      }
      event "Round T1 X": Value Change {
        n1030 = event-data() -> ()  [unwired: 7 out]
        n1031 = local read "BD 1 Frequency 1 (MHz)"() -> (w1386:dbl)
        n1032 = Round To Nearest(number=w1386) -> (nearest integer value=w1385:dbl)
        n1033 = property on="BD 1 Frequency 1 (MHz)" class="DigNum (strict)"("Val(Sgnl)"=w1385) -> ()  [unwired: 2 in, 2 out]
      }
      event "Round T2 X": Value Change {
        n1034 = event-data() -> ()  [unwired: 7 out]
        n1035 = local read "BD 1 Frequency 2 (MHz)"() -> (w1388:dbl)
        n1036 = Round To Nearest(number=w1388) -> (nearest integer value=w1387:dbl)
        n1037 = property on="BD 1 Frequency 2 (MHz)" class="DigNum (strict)"("Val(Sgnl)"=w1387) -> ()  [unwired: 2 in, 2 out]
      }
      event "Stop All": Value Change {
        n1038 = event-data() -> ()  [unwired: 7 out]
        n1039 = local read "Stop All"() -> (w1390:bool)
      }
      event "Delayed Interlace Start": Value Change {
        n1040 = event-data() -> ()  [unwired: 7 out]
        n1041 = flat-sequence {
          frame #0 {
            n1042 = Multiply(x="Delay to Interlace (s)", y=1000.0) -> (x*y=w1393:dbl)
            n1043 = Wait (ms)(milliseconds to wait=w1393) -> ()  [unwired: 1 out]
          }
          frame #1 {
            n1044 = property on="Laser interlacing mode (all lasers)" class="RadioBtnsControl (strict)"("Val(Sgnl)"=enum32{"Laser ON", "Laser OFF", "Interlace"}."Interlace" ("Value (Signaling)")) -> ()  [unwired: 2 in, 2 out]
          }
        }
      }
      event "BD 1 Amplitude 1 (%)", "BD 1 Amplitude 2 (%)", "BD 1 Amplitude 3 (%)", "BD 2 Amplitude 1 (%)", "BD 2 Amplitude 2 (%)", "BD 2 Amplitude 3 (%)", "Trap 1 ON", "Trap 2 ON", "Trap 3 ON", "Feedback On/Off", "All FB On/Off": Value Change {
        w1417 = i16 1 ("f")
        n1045 = event-data() -> ()  [unwired: 7 out]
        n1046 = local write "Trap 1 (ON/OFF)"("Trap 1 ON") -> ()
        n1047 = local write "Trap 2 (ON/OFF)"("Trap 2 ON") -> ()
        n1048 = Boolean To (0,1)(Boolean="Trap 3 ON") -> (0, 1=w1418:i16)
        n1049 = Boolean To (0,1)(Boolean="Trap 1 ON") -> (0, 1=w1419:i16)
        n1050 = Boolean To (0,1)(Boolean="Trap 2 ON") -> (0, 1=w1420:i16)
        n1051 = Select(t=w1420, s="Trap ON/OFF X or Y Amp?", f=w1417) -> (s? t:f=w1415:i16)
        n1052 = Select(t=w1419, s="Trap ON/OFF X or Y Amp?", f=w1417) -> (s? t:f=w1416:i16)
        n1053 = Select(t=w1418, s="Trap ON/OFF X or Y Amp?", f=w1417) -> (s? t:f=w1414:i16)
        n1054 = Select(t=w1417, s="Trap ON/OFF X or Y Amp?", f=w1420) -> (s? t:f=w1412:i16)
        n1055 = Select(t=w1417, s="Trap ON/OFF X or Y Amp?", f=w1419) -> (s? t:f=w1413:i16)
        n1056 = Select(t=w1417, s="Trap ON/OFF X or Y Amp?", f=w1418) -> (s? t:f=w1411:i16)
        n1057 = And(x="All FB On/Off", y="Feedback On/Off") -> (x .and. y?=w1409:cluster{"Set 1":bool, "Set 2":bool})
        n1058 = local read "BD 1 Amplitude 1 (%)"() -> (w1429:dbl)
        n1059 = local read "BD 1 Amplitude 2 (%)"() -> (w1428:dbl)
        n1060 = local read "BD 1 Amplitude 3 (%)"() -> (w1427:dbl)
        n1061 = Unbundle By Name(w1409) -> ("Set 1"=w1404:bool, "Set 2"=w1401:bool)
        n1062 = local read "Y RF Amplitude Limits (%)"() -> (w1397:T17)
        n1063 = local read "X RF Amplitude Limits (%)"() -> (w1398:T17)
        n1064 = local read "BD 2 Amplitude 1 (%)"() -> (w1430:dbl)
        n1065 = local read "BD 2 Amplitude 2 (%)"() -> (w1431:dbl)
        n1066 = local read "BD 2 Amplitude 3 (%)"() -> (w1432:dbl)
        n1067 = And(x="Trap 2 ON", y=w1401) -> (x .and. y?=w1399:bool)
        n1068 = And(x="Trap 1 ON", y=w1404) -> (x .and. y?=w1402:bool)
